vi "LoadProfileInfo.vi"(8 "error in (no error)":errorcluster, 11 "DataPatientPath":path) -> (0 "error out":errorcluster, 1 "Doctor":string, 2 "Operator":string, 3 "Name":string, 5 "Comment":string)   [LabVIEW 2013, in "main.lvlib"]
uses:
  main.lvlib
  <userlib>/_OpenG.lib/file/file.llb/File Exists - Scalar__ogtk.vi
  <vilib>/Utility/file.llb/Read From Spreadsheet File (string).vi
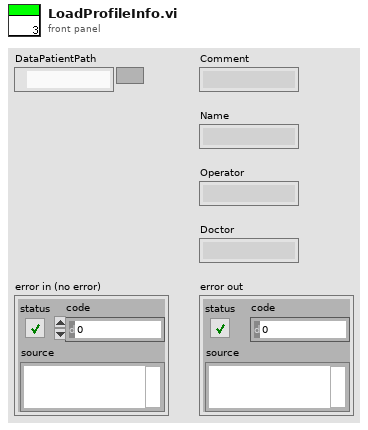
[diagram p1: front panel]
types:
  T1 = cluster{"id":string, "name":string, "operator":string, "doctor":string, "comment":string}
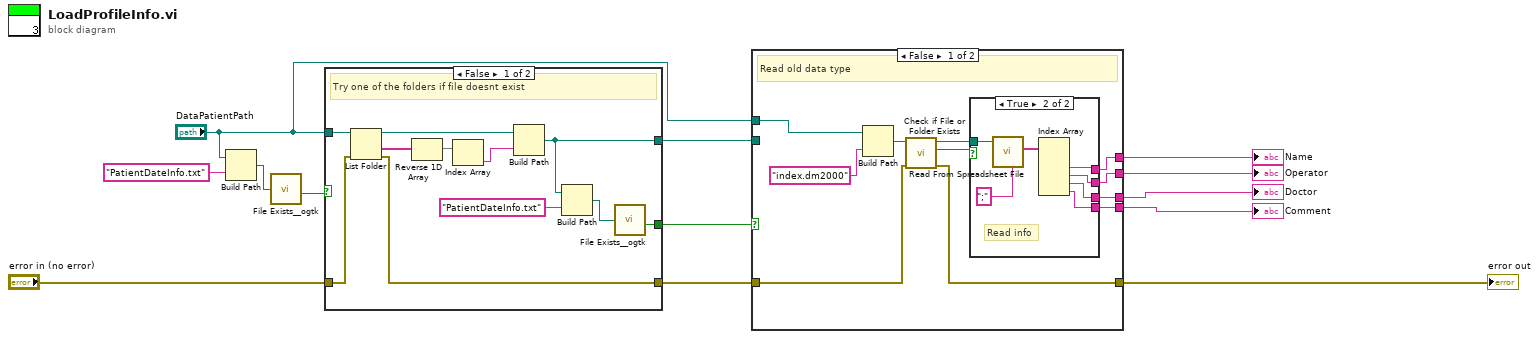
[diagram p0: block diagram]
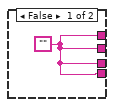
[diagram p3: hidden frame]
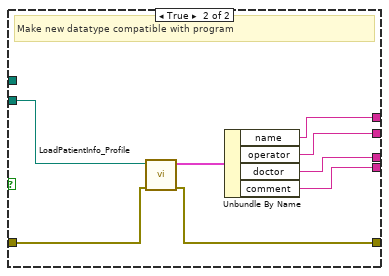
[diagram p4: hidden frame]
diagram:
  n1 = Build Path(base path="DataPatientPath", name or relative path="PatientDateInfo.txt") -> (appended path=w6:path)
  n2 = call-poly <userlib>:"File Exists__ogtk.vi"("file path"=w6) -> ("exists"=w2:bool)  [unwired: 6 in, 1 out]
  n3 = case shown="False" w2 {
    selector: w2 -> [_ w26]
    tunnel: [w22 w26] -> w8
    tunnel: "DataPatientPath" -> [w21 w27]
    tunnel: "error in (no error)" -> [w20 w25]
    tunnel: [w19 w25] -> w4
    tunnel: [w18 w27] -> w3
    frame False {
      # "Try one of the folders if file doesnt exist"
      n4 = List Folder(path=w21, error in=w20) -> (path out=w17:path, folder names=w14:string[], error out=w19:errorcluster)  [unwired: 2 in, 1 out]
      n5 = Reverse 1D Array(array=w14) -> (reversed array=w15:string[])
      n6 = Index Array(array=w15) -> (element=w16:string)  [unwired: 1 in]
      n7 = Build Path(base path=w17, name or relative path=w16) -> (appended path=w18:path)
      n8 = Build Path(base path=w18, name or relative path="PatientDateInfo.txt") -> (appended path=w23:path)
      n9 = call-poly <userlib>:"File Exists__ogtk.vi"("file path"=w23) -> ("exists"=w22:bool)  [unwired: 6 in, 1 out]
    }
    frame True {
    }
  }
  n10 = case shown="False" w8 {
    tunnel: [w38 w53] -> w13
    tunnel: w4 -> [w37 w54]
    tunnel: [w36 w48] -> w12
    tunnel: [w35 w49] -> w11
    tunnel: [w34 w50] -> w10
    tunnel: [w33 w51] -> w9
    tunnel: w3 -> [_ w47]
    tunnel: "DataPatientPath" -> [w28 _]
    frame False {
      # "Read old data type"
      n11 = Build Path(base path=w28, name or relative path="index.dm2000") -> (appended path=w30:path)
      n12 = call <vilib>:"Check if File or Folder Exists.vi"("error in (no error)"=w37, "path"=w30) -> ("error out"=w38:errorcluster, "file or folder exists?"=w32:bool, "dup path"=w31:path)  [unwired: 7 in]
      n13 = case shown="True" w32 {
        tunnel: w31 -> [_ w46]
        tunnel: [w39 w43] -> w33
        tunnel: [w39 w42] -> w34
        tunnel: [w39 w41] -> w35
        tunnel: [w39 w40] -> w36
        frame False {
          w39 = ""
        }
        frame True {
          # "Read info"
          n14 = call-poly <vilib>:"Read From Spreadsheet File.vi"("delimiter (\\t)"=";" ("delimiter (\\t)"), "file path (dialog if empty)"=w46) -> ("first row"=w45:string[])  [unwired: 5 in, 4 out]
          n15 = Index Array(array=w45) -> (element #2=w43:string, element #3=w42:string, element #4=w41:string, element #5=w40:string)  [unwired: 5 in, 1 out]
        }
      }
    }
    frame True {
      # "Make new datatype compatible with program"
      n16 = call "LoadPatientInfo_Profile.vi"("error in"=w54, "DataPatientPath"=w47) -> ("error out"=w53:errorcluster, "profile"=w52:T1)  [unwired: 8 in]
      n17 = Unbundle By Name(w52) -> ("name"=w51:string, "operator"=w50:string, "doctor"=w49:string, "comment"=w48:string)
    }
  }
  "error out" <- w13
  "Comment" <- w12
  "Doctor" <- w11
  "Operator" <- w10
  "Name" <- w9
